vi "basic_gpib_write_and_read.vi"() -> ()   [LabVIEW 2013]
doc: "This VI performs simple GPIB VISA communication with a GPIB instrument. It will send the user specified command and return a number of bytes equal or less than the byte count specified. The program default values may work with the instrument(s), but complete the following steps to ensure the program will run properly:\n1. Make sure your instrument(s) show up in Measurement and Automation Explorer (MAX).\n2. In the VISA resource name dropdown box, select your instrument.\n3. Ensure the instrument address is correct.\n4. Type in a known command for the instrument in the \"Write Buffer\" field.\n5. Type in the byte count expected from the instrument after sending the command in the \"Write Buffer\" field.\n6. Type in the wait needed for the instrument to respond to the command.\n7. Power cycle the instrument to ensure it is ready to receive commands.\n8. Run the program."
panel:
  in  "VISA Resource Name":refnum<visa-resource-name>="GPIB0::2::INSTR"
  in  "Milliseconds to Wait":u32=50
  out "Read Buffer":string
  in  "Byte Count":u32=100
  in  "Write Buffer":string="*IDN?"
  # "Select Help»Show Context Help and move the cursor \nover the VI icon to display help for this VI."
  # "GPIB Instrument\nAddress"
  # "Command to Send \nto Instrument"
  # "Byte Count to\nRead from Instrument"
  # "Wait between Write\nand Read"
  # "Return Value from \nInstrument"
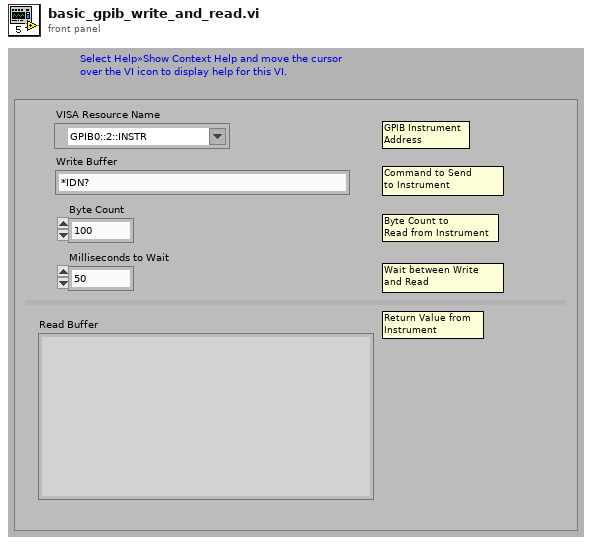
[diagram p1: front panel]
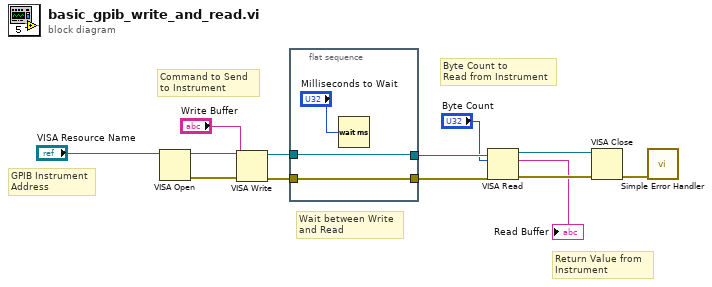
[diagram p0: block diagram]
diagram:
  # "Wait between Write\nand Read"
  # "Return Value from \nInstrument"
  # "Byte Count to\nRead from Instrument"
  # "Command to Send \nto Instrument"
  # "GPIB Instrument\nAddress"
  n1 = VISA Open(VISA resource name="VISA Resource Name") -> (VISA resource name=w12:refnum<visa-resource-name>, error out=w10:errorcluster)  [unwired: 4 in]
  n2 = VISA Write(VISA resource name=w12, write buffer="Write Buffer", error in (no error)=w10) -> (VISA resource name out=w5:refnum<visa-resource-name>, error out=w4:errorcluster)  [unwired: 1 out]
  n3 = flat-sequence {
    tunnel: [w15] -> w2
    tunnel: w5 -> [w15]
    tunnel: [w14] -> w3
    tunnel: w4 -> [w14]
    frame #0 {
      n4 = Wait (ms)(milliseconds to wait="Milliseconds to Wait") -> ()  [unwired: 1 out]
    }
  }
  n5 = VISA Read(VISA resource name=w2, byte count="Byte Count", error in (no error)=w3) -> (VISA resource name out=w11:refnum<visa-resource-name>, read buffer=→"Read Buffer":string, error out=w9:errorcluster)  [unwired: 1 out]
  n6 = VISA Close(VISA resource name=w11, error in (no error)=w9) -> (error out=w8:errorcluster)
  n7 = call <vilib>:"Simple Error Handler.vi"("error in (no error)"=w8) -> ()  [unwired: 4 in, 5 out]
